vi "Write subpanel ref.vi"(8 "error in (no error)":errorcluster, 10 "subpanel_ref":refnum<vi>, 11 "View Cfg Base Template in":refnum<class "[V] Sys Cfg Base.lvclass">) -> (0 "error out":errorcluster, 3 "View Cfg Base Template out":refnum<class "[V] Sys Cfg Base.lvclass">)   [LabVIEW 2023]
uses:
  [V] Sys Cfg Base.lvclass
  C:/Program Files (x86)/National Instruments/LabVIEW 2023/vi.lib/ActorFramework/Actor/Actor.lvclass
  D:/03 GitHub/LabVIEW-System-Config/[V] Sys Cfg Base/[V] Sys Cfg Base/[V] Sys Cfg Base.lvclass
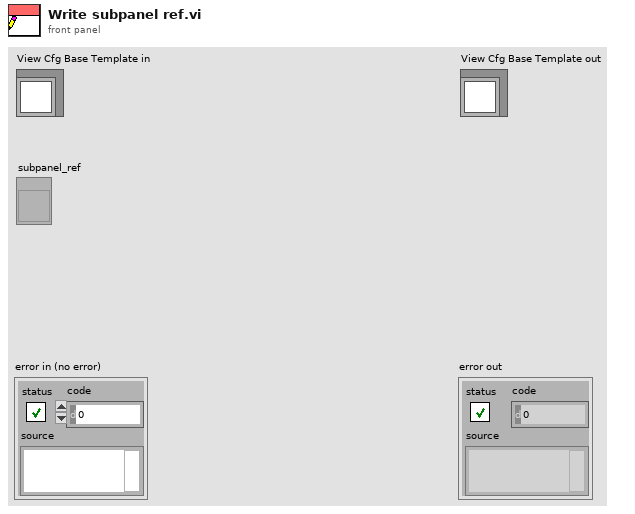
[diagram p1: front panel]
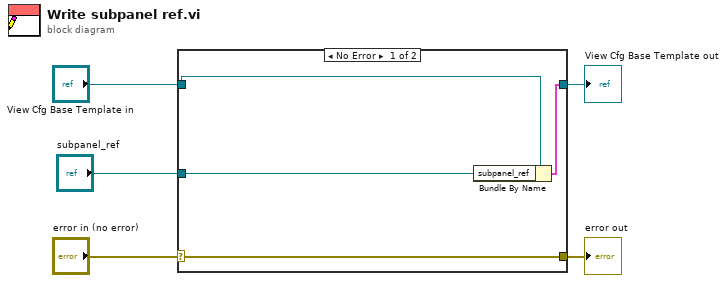
[diagram p0: block diagram]
diagram:
  n1 = case shown="No Error" "error in (no error)" {
    selector: "error in (no error)" -> [w9 w10]
    tunnel: [w9 w10] -> w4
    tunnel: [w7 w11] -> w2
    tunnel: "View Cfg Base Template in" -> [w8 w11]
    tunnel: "subpanel_ref" -> [w6 _]
    frame No Error {
      n2 = Bundle By Name(cluster=w8, "subpanel_ref"=w6) -> (w7:cluster{})
    }
    frame Error {
    }
  }
  "error out" <- w4
  "View Cfg Base Template out" <- w2
